vi "Handle Heartbeat Message.vi"(8 "error in":errorcluster, 10 "CANopen Message":refnum<class "CANopen Response Message.lvclass">, 11 "CANopen Master in":refnum<class "CANopen Master.lvclass">) -> (0 "error out":errorcluster, 3 "CANopen Master out":refnum<class "CANopen Master.lvclass">)   [LabVIEW 2024, in "CANopen Master.lvlib" / "CANopen Master.lvclass"]
doc: "Handles a received NMT Message. Resets an awaited heartbeat. Extracts Sender's state and fires a Node Discovered event in case a new node is on the bus."
uses:
  CANopen Master.lvclass
  CANopen Response/CANopen Response Message.lvclass
  CANopen Master.lvclass/CANopen Master.ctl
  Heartbeat/Heartbeat.lvclass
  Network Mangement/Network Mangement.lvclass
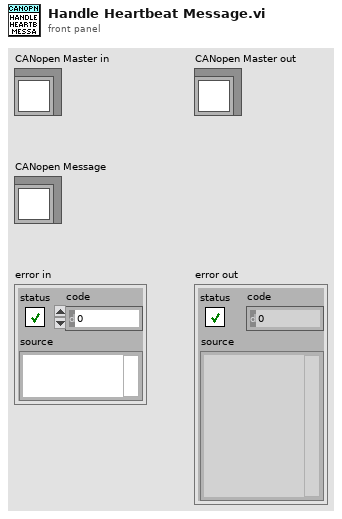
[diagram p1: front panel]
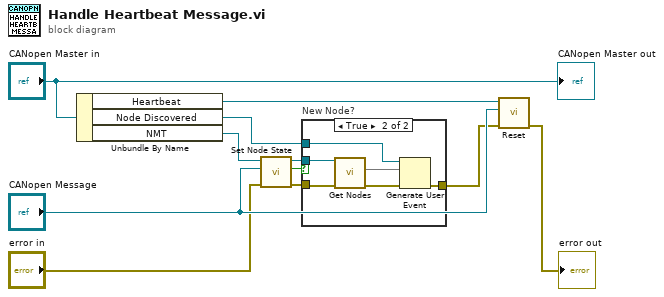
[diagram p0: block diagram]
diagram:
  n1 = Unbundle By Name("CANopen Master in") -> ("Heartbeat"=w10:refnum<class "Heartbeat.lvclass">, "Node Discovered"=w2:refnum<user-event>, "NMT"=w3:refnum<class "Network Mangement.lvclass">)
  n2 = call "Set Node State.vi"("Error In"="error in", "CANopen Message"="CANopen Message", "reference in"=w3) -> ("Error Out"=w5:errorcluster, "New Node/State?"=w6:bool, "reference out"=w4:refnum<class "Network Mangement.lvclass">)  [unwired: 6 in]
  n3 = case "New Node?" shown="True" w6 {
    tunnel: w5 -> [w12 w17]
    tunnel: w4 -> [_ w18]
    tunnel: w2 -> [_ w15]
    tunnel: [w12 w13] -> w1
    frame False {
    }
    frame True {
      n4 = call "Get Nodes.vi"("Error In"=w17, "reference in"=w18) -> ("Error Out"=w14:errorcluster, "Nodes"=w16:map{u8, u8})  [unwired: 7 in, 1 out]
      n5 = Generate User Event(user event=w15, event data cluster=w16, error in=w14) -> (error out=w13:errorcluster)  [unwired: 1 in, 1 out]
    }
  }
  n6 = call "Reset.vi"("Error In"=w1, "CANopen Message"="CANopen Message", "reference in"=w10) -> ("Error Out"=→"error out":errorcluster)  [unwired: 7 in, 1 out]
  "CANopen Master out" <- "CANopen Master in"
